vi "lab4_task1.vi"() -> ()   [LabVIEW 2021]
uses:
  <vilib>/express/express analysis/Spectral/Block/exnSpectralBlock spectral measurements PSD poly.vi
  <vilib>/express/express analysis/Spectral/Block/exnSpectralBlock spectral measurements PSD DDT.vi
  <vilib>/express/express analysis/Spectral/XNode/ExpressSpectralMeasurementsBlockNode.xnode
  <vilib>/Analysis/NI_AALPro.lvlib
panel:
  out "number samples":dbl
  in  "Duration":dbl=10000.0
  in  "Sampling rate":dbl=10000.0
  out "Intensity Chart":dbl[][](graph)
  out "Power spectral density":dynamicdata(graph)
  in  "# bins":i32
  out "Histogram Graph":T1(graph)
  out "rms":dbl
  out "peak to peak":dbl
  out "mean":dbl
  out "data":dynamicdata(graph)
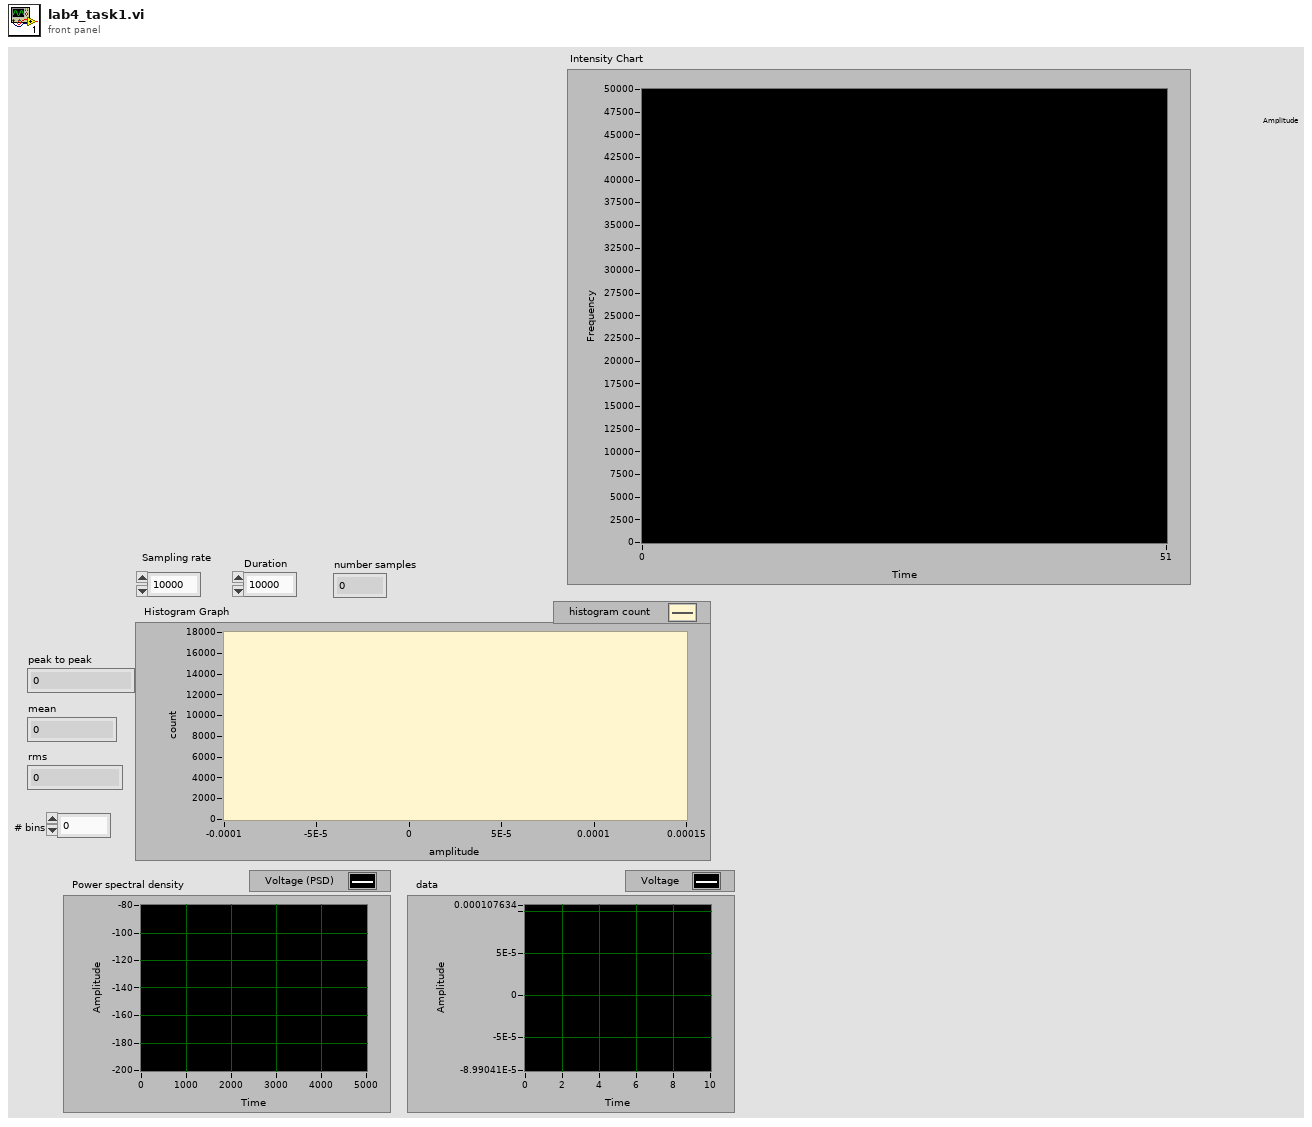
[diagram p1: front panel]
types:
  T1 = cluster{"X Values":dbl[], "Histogram: h(x)":i32[]}
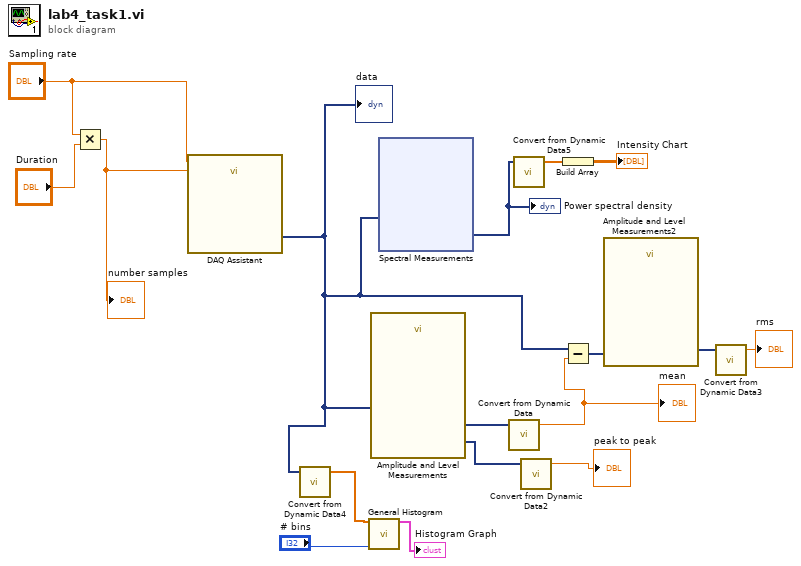
[diagram p0: block diagram]
diagram:
  n1 = Multiply(x="Sampling rate", y="Duration") -> (x*y=w1:dbl)
  "number samples" <- w1
  n2 = call "DAQ Assistant"("rate"="Sampling rate", "number of samples"=w1) -> ("data"=w7:dynamicdata)  [unwired: 15 in, 2 out]
  "data" <- w7
  n3 = call "Convert from Dynamic Data4"("Dynamic Data Type"=w7) -> ("Array"=w8:dbl[])  [unwired: 3 in]
  n4 = call <vilib>:"General Histogram.vi"("X"=w8, "# bins"="# bins") -> ("Histogram Graph"=→"Histogram Graph":T1)  [unwired: 9 in, 4 out]
  n5 = call "Amplitude and Level Measurements"("Signals"=w7) -> ("Mean (DC)"=w17:dynamicdata, "Peak to Peak"=w16:dynamicdata)  [unwired: 12 in, 1 out]
  n6 = xnode "Spectral Measurements"("Signals"=w7) -> ("PSD"=w6:dynamicdata)  [unwired: 1 in, 1 out]
  "Power spectral density" <- w6
  n7 = call "Convert from Dynamic Data"("Dynamic Data Type"=w17) -> ("Scalar"=w14:dbl)  [unwired: 3 in]
  "mean" <- w14
  n8 = call "Convert from Dynamic Data5"("Dynamic Data Type"=w6) -> ("Array"=w5:dbl[])  [unwired: 3 in]
  n9 = call "Convert from Dynamic Data2"("Dynamic Data Type"=w16) -> ("Scalar"=→"peak to peak":dbl)  [unwired: 3 in]
  n10 = Build Array(w5) -> (→"Intensity Chart":dbl[][])
  n11 = Subtract(x=w7, y=w14) -> (x-y=w13:dynamicdata)
  n12 = call "Amplitude and Level Measurements2"("Signals"=w13) -> ("RMS"=w12:dynamicdata)  [unwired: 13 in, 1 out]
  n13 = call "Convert from Dynamic Data3"("Dynamic Data Type"=w12) -> ("Scalar"=→"rms":dbl)  [unwired: 3 in]
